vi "AVT Pike.vi"() -> ()   [LabVIEW 2011]
uses:
  <vilib>/vision/driver/NI_Vision_Acquisition_Software.lvlib
panel:
  in  "stop":bool
  out "acquired FPS":dbl
  out "error out":errorcluster
  in  "error in":errorcluster
  out "Video":dbl[][](graph)
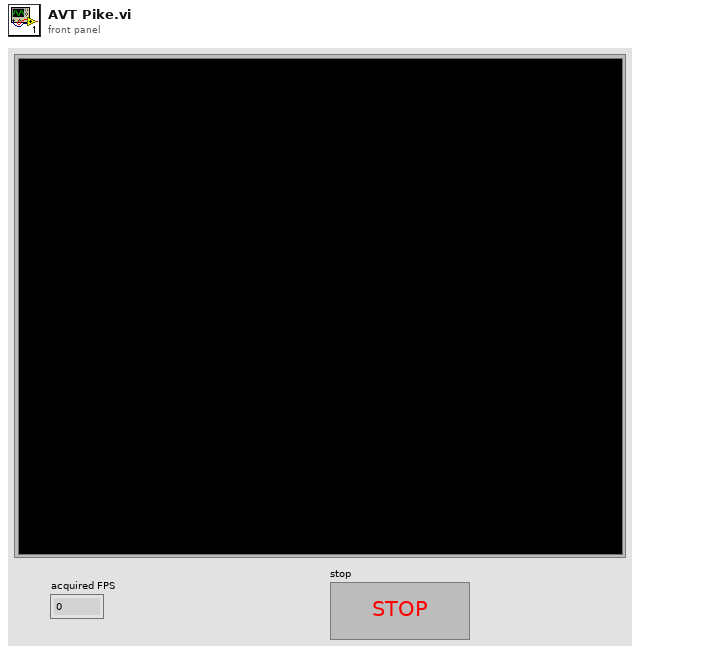
[diagram p1: front panel]
types:
  T1 = typedef "Image Type" = u32
  T2 = typedef "IMAQdx.ctl" = refnum<k21>
  T3 = typedef "IMAQ Image.ctl" = refnum<image>
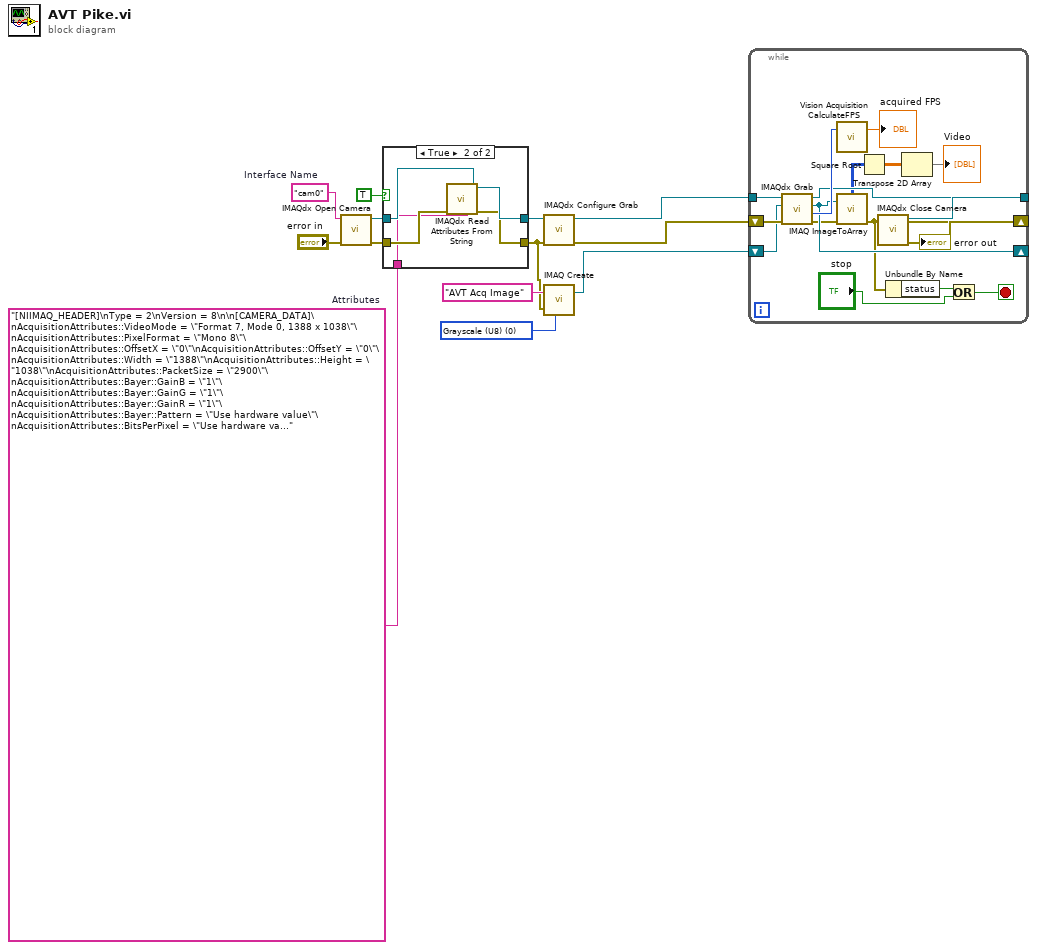
[diagram p0: block diagram]
diagram:
  w2 = "[NIIMAQ_HEADER]\nType = 2\nVersion = 8\n\n[CAMERA_DATA]\nAcquisitionAttributes::VideoMode = \"Format 7, Mode 0, 1388 x 1038\"\nAcquisitionAttributes::PixelFormat = \"Mono 8\"\nAcquisitionAttributes::OffsetX = \"0\"\nAcquisitionAttributes::OffsetY = \"0\"\nAcquisitionAttributes::Width = \"1388\"\nAcquisitionAttributes::Height = \"1038\"\nAcquisitionAttributes::PacketSize = \"2900\"\nAcquisitionAttributes::Bayer::GainB = \"1\"\nAcquisitionAttributes::Bayer::GainG = \"1\"\nAcquisitionAttributes::Bayer::GainR = \"1\"\nAcquisitionAttributes::Bayer::Pattern = \"Use hardware value\"\nAcquisitionAttributes::BitsPerPixel = \"Use hardware value\"\nAcquisitionAttributes::Controller::DesiredStreamChannel = \"0\"\nAcquisitionAttributes::Controller::StreamChannelMode = \"Automatic\"\nAcquisitionAttributes::IgnoreFirstFrame = \"false\"\nAcquisitionAttributes::OverwriteMode = \"Get Newest\"\nAcquisitionAttributes::PixelSignedness = \"Signed\"\nAcquisitionAttributes::ReceiveTimestampMode = \"None\"\nAcquisitionAttributes::ReserveDualPackets = \"false\"\nAcquisitionAttributes::ShiftPixelBits = \"true\"\nAcquisitionAttributes::Speed = \"800 Mbps\"\nAcquisitionAttributes::SwapPixelBytes = \"false\"\nAcquisitionAttributes::Timeout = \"5000\"\nCameraAttributes::AutoExposure::Mode = \"Relative\"\nCameraAttributes::Brightness::Mode = \"Relative\"\nCameraAttributes::Gain::Mode = \"Auto\"\nCameraAttributes::Gamma::Mode = \"Off\"\nCameraAttributes::Shutter::Mode = \"Relative\"\nCameraAttributes::TriggerDelay::Mode = \"Off\"\nCameraAttributes::AutoExposure::Value = \"125\"\nCameraAttributes::Brightness::Value = \"16\"\nCameraAttributes::Gain::Value = \"0\"\nCameraAttributes::Shutter::Value = \"2000\"\nCameraAttributes::Trigger::TriggerMode = \"Off\"\nCameraAttributes::Trigger::TriggerActivation = \"Level Low\"\nCameraAttributes::Trigger::TriggerParameter = \"0\"\n"  # Attributes
  w3 = T1 0 items=["Grayscale (U8)", "Grayscale (I16)", "Grayscale (SGL)", "Complex (CSG)", "RGB (U32)", "HSL (U32)", "RGB (U64)", "Grayscale (U16)"] ("Image Type")
  w14 = "cam0"  # Interface Name
  n1 = call <vilib>:"IMAQdx Open Camera.vi"("error in"="error in", "Session In"=w14) -> ("error out"=w7:errorcluster, "Session Out"=w8:T2)  [unwired: 1 in, 7 out]
  n2 = case shown="True" TRUE ("Init Attributes") {
    tunnel: w8 -> [w18 w23]
    tunnel: w7 -> [w17 w22]
    tunnel: [w18 w21] -> w6
    tunnel: [w17 w20] -> w1
    tunnel: w2 -> [_ w19]
    frame False {
    }
    frame True {
      n3 = call <vilib>:"IMAQdx Read Attributes From String.vi"("error in"=w22, "Attributes String In"=w19, "Session In"=w23) -> ("error out"=w20:errorcluster, "Session Out"=w21:T2)  [unwired: 7 out]
    }
  }
  n4 = call <vilib>:"IMAQdx Configure Grab.vi"("error in"=w1, "Session In"=w6) -> ("error out"=w15:errorcluster, "Session Out"=w12:T2)  [unwired: 8 out]
  n5 = call "IMAQ Create"("Image Name"="AVT Acq Image", "Image Type"=w3, "error in (no error)"=w1) -> ("New Image"=w13:T3)  [unwired: 1 in, 2 out]
  n6 = while {
    tunnel: w12 -> [w34]
    tunnel: [w33] -> w10
    shift-right: [w26] -> w11
    shift-left: w15 -> [w38]
    shift-right: [w29] -> _
    shift-left: w13 -> [w35]
    stop <- w30 stop-if-true
    n7 = call <vilib>:"IMAQdx Grab.vi"("error in"=w38, "Image In"=w35, "Session In"=w34) -> ("error out"=w27:errorcluster, "Buffer Number Out"=w36:u32, "Image Out"=w29:T3, "Session Out"=w33:T2)  [unwired: 1 in, 4 out]
    n8 = call <vilib>:"Vision Acquisition CalculateFPS.vi"("buffer number"=w36) -> ("acquired FPS"=→"acquired FPS":dbl)  [unwired: 2 out]
    n9 = call "IMAQ ImageToArray"("error in (no error)"=w27, "Image"=w29) -> ("error out"=w26:errorcluster, "Image Pixels (U8)"=w28:u8[][])  [unwired: 2 in, 3 out]
    n10 = Square Root(x=w28) -> (sqrt(x)=w25:dbl[][])
    n11 = Unbundle By Name(w26) -> ("status"=w37:bool)
    n12 = Transpose 2D Array(2D array=w25) -> (transposed array=→"Video":dbl[][])
    n13 = Or(x=w37, y="stop") -> (x .or. y?=w30:bool)
  }
  n14 = call <vilib>:"IMAQdx Close Camera.vi"("error in"=w11, "Session In"=w10) -> ("error out"=→"error out":errorcluster)  [unwired: 9 out]
